vi "KeithMeasFrequency.vi"() -> ()   [LabVIEW 2017]
uses:
  <vilib>/Instr/_visa.llb/GPIB Status Boolean Array.ctl
panel:
  in  "milliseconds to wait":u32
  out "frequency":dbl
  out "query 2":string
  in  "Command 2":string
  out "ibsta 2":T1
  out "ibsta":T1
  out "error out":errorcluster
  out "query 1":string
  in  "Command 1":string
  in  "mode":i16
  in  "address":i16=16
  in  "bus":i32
  in  "Number of loopy loops":i32
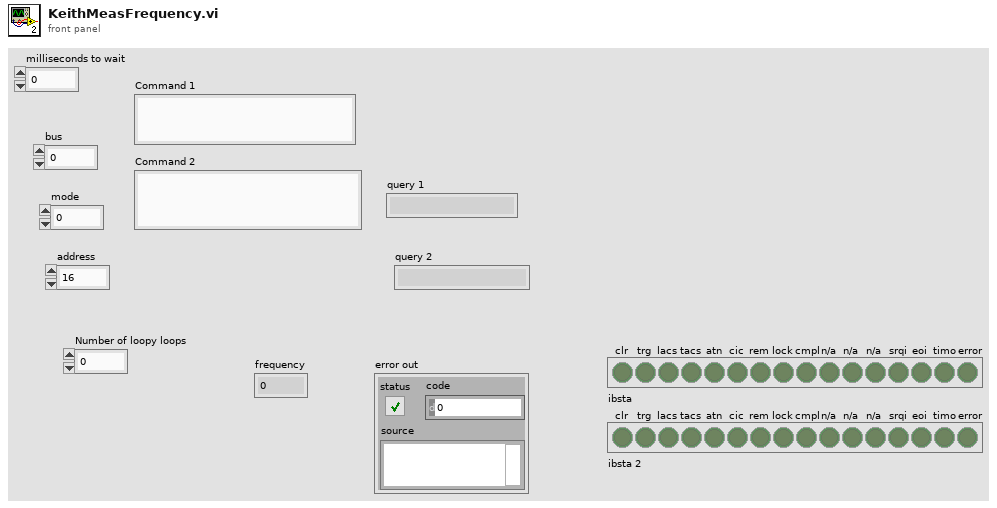
[diagram p1: front panel]
types:
  T1 = typedef "GPIB Status Boolean Array.ctl" = bool[]
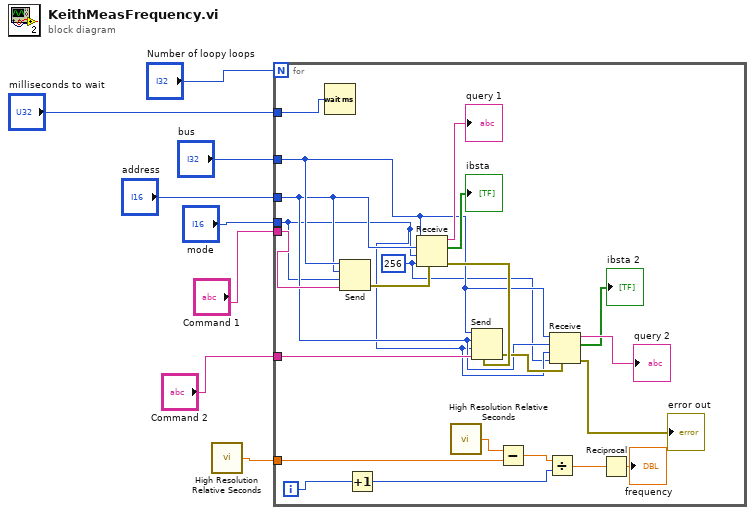
[diagram p0: block diagram]
diagram:
  n1 = call <vilib>:"High Resolution Relative Seconds.vi"() -> ("relative seconds"=w2:dbl)
  n2 = for {
    N: "Number of loopy loops" -> [_]
    tunnel: "Command 1" -> [w28]
    tunnel: "mode" -> [w19]
    tunnel: "address" -> [w20]
    tunnel: "bus" -> [w21]
    tunnel: "Command 2" -> [w26]
    tunnel: w2 -> [w15]
    tunnel: "milliseconds to wait" -> [w9]
    i -> [w11]
    w18 = 256 ("count")
    n3 = Wait (ms)(milliseconds to wait=w9) -> ()  [unwired: 1 out]
    n4 = Send(0:w21, 2:w20, 3:w19, 5:w28) -> (8:w30:errorcluster)  [unwired: 1 in, 2 out]
    n5 = Increment(x=w11) -> (x+1=w10:i32)
    n6 = Receive(4:w30, 6:w18, 7:w19, 8:w20, 9:w21) -> (0:w24:errorcluster, 2:→"ibsta":bool[], 3:→"query 1":string)  [unwired: 1 out]
    n7 = call <vilib>:"High Resolution Relative Seconds.vi"() -> ("relative seconds"=w16:dbl)
    n8 = Send(0:w21, 2:w20, 3:w19, 4:w24, 5:w26) -> (8:w23:errorcluster)  [unwired: 2 out]
    n9 = Subtract(x=w16, y=w15) -> (x-y=w13:dbl)
    n10 = Divide(x=w13, y=w10) -> (x/y=w14:dbl)
    n11 = Receive(4:w23, 6:w18, 7:w19, 8:w20, 9:w21) -> (0:→"error out":errorcluster, 2:→"ibsta 2":bool[], 3:→"query 2":string)  [unwired: 1 out]
    n12 = Reciprocal(x=w14) -> (1/x=→"frequency":dbl)
  }
